vi "Open VI Ref from Path.vi"(8 "error in":errorcluster, 10 "VI Path":path) -> (0 "error out":errorcluster, 2 "VI Ref":refnum<vi>)   [LabVIEW 2016, in "Flex UI.lvclass"]
uses:
  Flex UI.lvclass
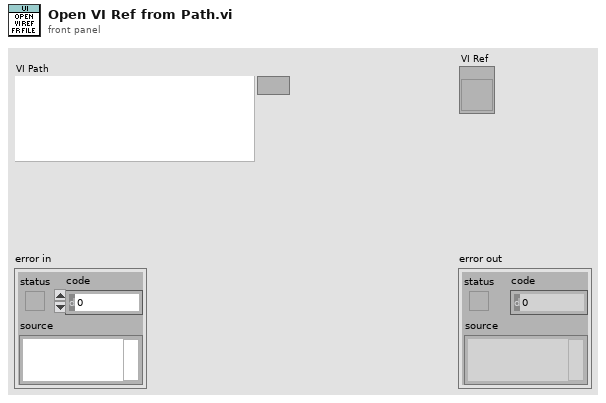
[diagram p1: front panel]
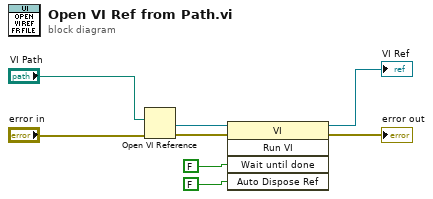
[diagram p0: block diagram]
diagram:
  n1 = Open VI Reference(vi path="VI Path", error in (no error)="error in") -> (vi reference=w4:refnum<vi>, error out=w5:errorcluster)  [unwired: 4 out]
  n2 = invoke on="Invoke Node" class="VI" method="Run VI"(reference=w4, error in=w5, "Wait until done"=FALSE ("Wait Until Done"), "Auto Dispose Ref"=FALSE ("Auto Dispose Reference")) -> (reference out=→"VI Ref":refnum<vi>, error out=→"error out":errorcluster)  [unwired: 1 in, 3 out]
